vi "SetHigherBound.vi"(8 "error in":errorcluster, 10 "HigherBond":dbl, 11 "RealMeasureLimit in":refnum<class "RealMeasureLimit.lvclass">) -> (0 "error out":errorcluster, 3 "RealMeasureLimit out":refnum<class "RealMeasureLimit.lvclass">)   [LabVIEW 2021, in "ProligentXMLGenerator.lvlib" / "RealMeasureLimit.lvclass"]
doc: "Real Measure Limit Higher Bound"
uses:
  RealMeasureLimit.lvclass
  RealMeasureLimit.lvclass/RealMeasureLimit.ctl
  RangeMeasureLimit/RangeMeasureLimit.lvclass
  Base/Decimal/Decimal.lvclass
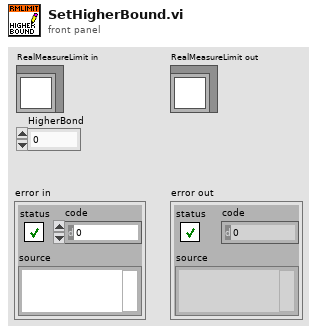
[diagram p1: front panel]
types:
  T1 = typedef "ProligentXMLGenerator.lvlib/RealMeasureLimit.lvclass/Data.ctl" = cluster{"LowerBound":refnum<class "Decimal.lvclass">, "HigherBound":refnum<class "Decimal.lvclass">}
  T2 = typedef "ProligentXMLGenerator.lvlib/RangeMeasureLimit.lvclass/ComparisonType.ctl" = enum16{"LowerBound <= X <= HigherBound", "LowerBound < X <= HigherBound", "LowerBound <= X < HigherBound", "LowerBound < X < HigherBound", "LowerBound <= X", "LowerBound < X", "X <= HigherBound", "X < HigherBound", "X == HigherBound", "X != HigherBound", "X <= LowerBound OR HigherBound <= X", "X < LowerBound OR HigherBound <= X", "X <= LowerBound OR HigherBound < X", "X < LowerBound OR HigherBound < X"}
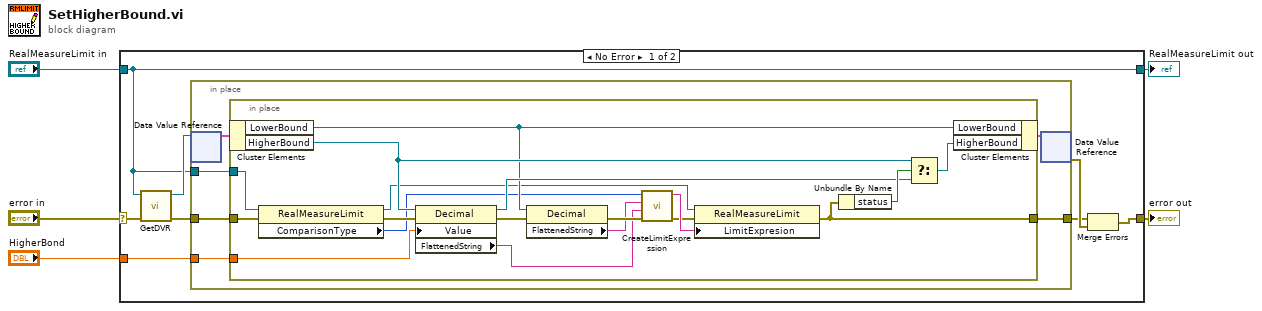
[diagram p0: block diagram]
diagram:
  n1 = case shown="No Error" "error in" {
    selector: "error in" -> [w7 w38]
    tunnel: "RealMeasureLimit in" -> [w6 w39]
    tunnel: [w12 w38] -> w2
    tunnel: "HigherBond" -> [w11 _]
    tunnel: [w6 w39] -> w1
    frame No Error {
      n2 = call "GetDVR.vi"("error in"=w7, "RealMeasureLimit"=w6) -> ("error out"=w10:errorcluster, "DVRReference"=w13:refnum<data-value>)  [unwired: 8 in]
      n3 = in-place "In Place Element Structure" {
        in-place-border: w11 -> [w19]
        in-place-border: w10 -> [w16]
        in-place-border: [w15] -> w8
        in-place-border: w6 -> [w14]
        n4 = in-place-dvr #1(w13) -> (w18:T1)  [unwired: 1 out]
        n5 = in-place "In Place Element Structure" {
          in-place-border: w19 -> [w31]
          in-place-border: w16 -> [w37]
          in-place-border: [w34] -> w15
          in-place-border: w14 -> [w22]
          n6 = in-place-cluster #2(w18) -> ("LowerBound"=w24:refnum<class "Decimal.lvclass">, "HigherBound"=w27:refnum<class "Decimal.lvclass">)
          n7 = property class="RealMeasureLimit"(reference=w22, error in=w37) -> (reference out=w21:refnum<class "RealMeasureLimit.lvclass">, error out=w23:errorcluster, "ComparisonType"=w20:T2)
          n8 = property class="Decimal"(reference=w27, error in=w23, "Value"=w31) -> (reference out=w25:refnum<class "Decimal.lvclass">, error out=w33:errorcluster, "FlattenedString"=w30:string)
          n9 = property class="Decimal"(reference=w24, error in=w33) -> (error out=w32:errorcluster, "FlattenedString"=w29:string)  [unwired: 1 out]
          n10 = call "CreateLimitExpression.vi"("error in"=w32, "HigherBound"=w30, "LowerBound"=w29, "ComparisonType"=w20) -> ("error out"=w35:errorcluster, "LimitExpression"=w36:string)  [unwired: 6 in]
          n11 = property class="RealMeasureLimit"(reference=w21, error in=w35, "LimitExpresion"=w36) -> (error out=w34:errorcluster)  [unwired: 1 out]
          n12 = Unbundle By Name(w34) -> ("status"=w26:bool)
          n13 = Select(t=w27, s=w26, f=w25) -> (s? t:f=w28:refnum<class "Decimal.lvclass">)
          n14 = in-place-cluster #2("LowerBound"=w24, "HigherBound"=w28) -> (w17:T1)
        }
        n15 = in-place-dvr #1(w17) -> (w9:errorcluster)  [unwired: 1 out]
      }
      n16 = Merge Errors(w8, w9) -> (w12:errorcluster)
    }
    frame Error {
    }
  }
  "error out" <- w2
  "RealMeasureLimit out" <- w1
